vi "Add SR Popup.vi"(8 "error in":errorcluster, 9 "Monitor":u16) -> (0 "error out":errorcluster, 2 "New SR?":bool, 3 "SR array out":i32[](array[numeric]))   [LabVIEW 2018]
uses:
  <vilib>/Utility/miscctls.llb/LVPointTypeDef.ctl
panel:
  in  "Close":bool
  in  "Add SR":bool
  in  "SR to Add":string
  # "Enter SR number(s) seperated by commas\n and press \"Add SRs\" to add it to the list"
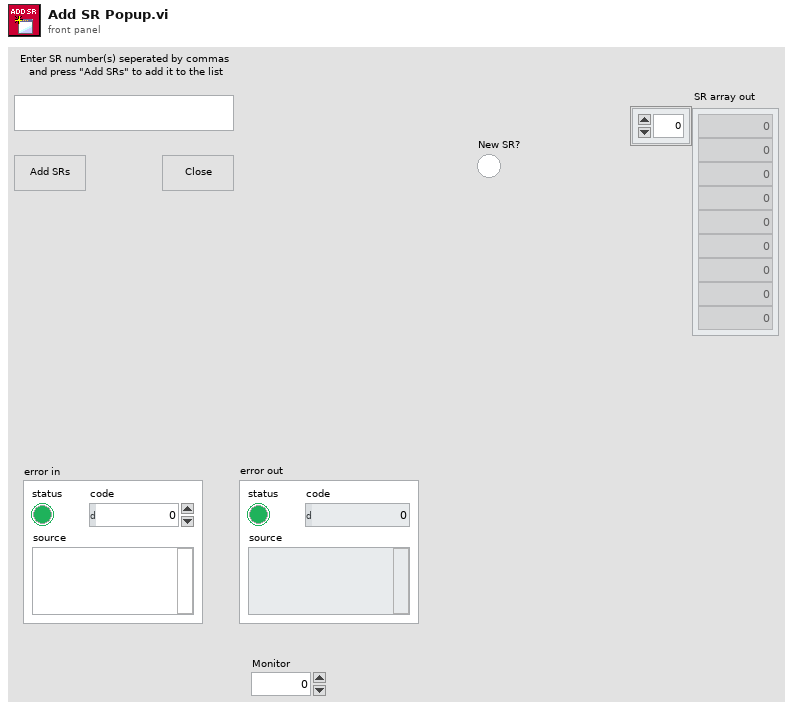
[diagram p1: front panel]
types:
  T1 = typedef "LVPointTypeDef.ctl" = cluster{"Horizontal":i16, "Vertical":i16}
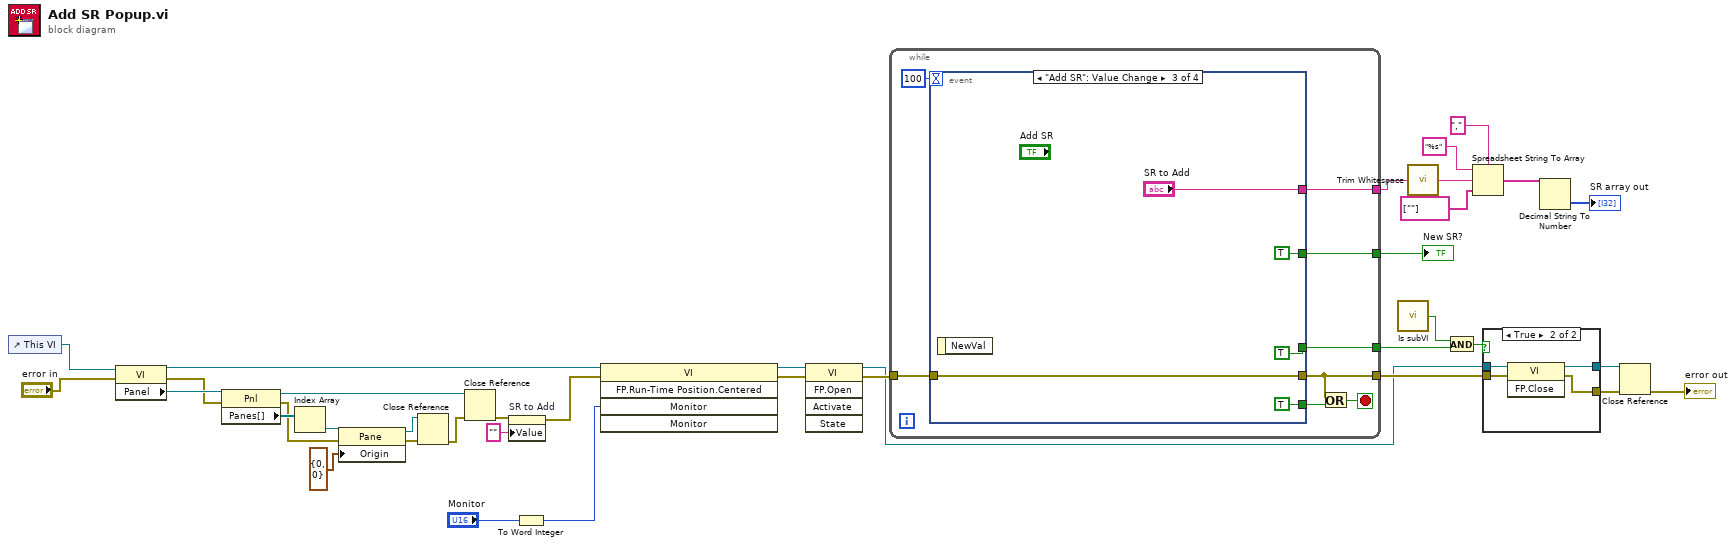
[diagram p0: block diagram]
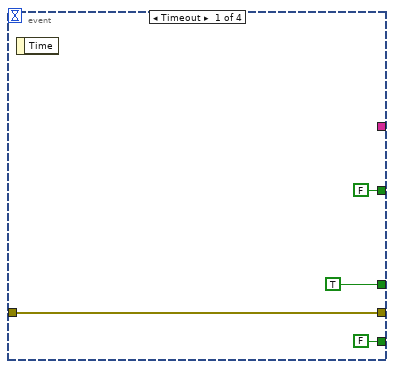
[diagram p3: hidden frame]
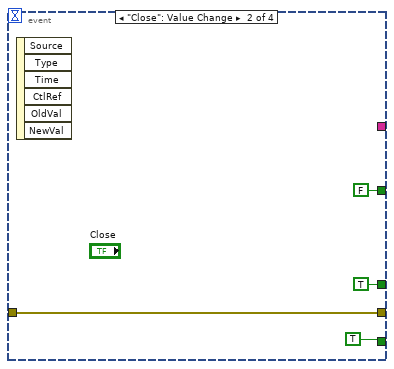
[diagram p4: hidden frame]
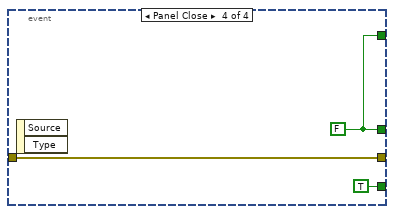
[diagram p5: hidden frame]
diagram:
  n1 = control-ref of="This VI"() -> (w12:refnum<vi>)
  n2 = property class="VI"(reference=w12, error in="error in") -> (reference out=w1:refnum<vi>, error out=w13:errorcluster, "Panel"=w14:refnum<vi>)
  n3 = property class="Pnl"(reference=w14, error in=w13) -> (reference out=w15:refnum<vi>, error out=w20:errorcluster, "Panes[]"=w22:refnum<vi>[])
  n4 = Index Array(array=w22) -> (element=w21:refnum<vi>)  [unwired: 1 in]
  n5 = property class="Pane"(reference=w21, error in=w20, "Origin"=T1 {"Horizontal"=0, "Vertical"=0}) -> (reference out=w18:refnum<vi>, error out=w17:errorcluster)
  n6 = Close Reference(reference=w18, error in (no error)=w17) -> (error out=w16:errorcluster)
  n7 = Close Reference(reference=w15, error in (no error)=w16) -> (error out=w8:errorcluster)
  n8 = property on="SR to Add" class="Str"(error in=w8, "Value"="" ("SR to Add")) -> (error out=w2:errorcluster)  [unwired: 1 in, 1 out]
  n9 = To Word Integer(number="Monitor") -> (16bit integer=w3:i16)
  n10 = invoke class="VI" method="FP.Run-Time Position.Centered"(reference=w1, error in=w2, "Monitor"=w3) -> (reference out=w6:refnum<vi>, error out=w5:errorcluster)  [unwired: 2 in, 3 out]
  n11 = invoke class="VI" method="FP.Open"(reference=w6, error in=w5) -> (reference out=w9:refnum<vi>, error out=w10:errorcluster)  [unwired: 3 in, 3 out]
  n12 = while {
    tunnel: w10 -> [w43]
    tunnel: [w41] -> w37
    tunnel: [w44] -> w24
    tunnel: [w39] -> w33
    tunnel: [w38] -> w31
    stop <- w42 stop-if-true
    n13 = event shown="[2] \"Add SR\": Value Change" {
      selector: _ -> [_ _ _ _]
      dyn-events: _ -> [_ _ _ _]
      timeout: 100 -> [_ _ _ _]
      tunnel: w43 -> [w48 w51 w58 w61]
      tunnel: [w48 w51 w58 w61] -> w41
      tunnel: [TRUE TRUE TRUE w59] -> w44
      tunnel: [FALSE TRUE TRUE TRUE] -> w40
      tunnel: [FALSE FALSE TRUE w59] -> w39
      tunnel: [_ _ "SR to Add" _] -> w38
      event Timeout {
        n14 = event-data() -> ()  [unwired: 1 in, 1 out]
      }
      event "Close": Value Change {
        n15 = event-data() -> ()  [unwired: 1 in, 6 out]
      }
      event "Add SR": Value Change {
        n16 = event-data() -> ()  [unwired: 1 in, 1 out]
      }
      event Panel Close {
        w59 = FALSE
        n17 = event-data() -> ()  [unwired: 1 in, 2 out]
      }
    }
    n18 = Or(x=w41, y=w40) -> (x .or. y?=w42:bool)
  }
  "New SR?" <- w33
  n19 = call "Is subVI.vi"() -> ("Is subVI?"=w23:bool)  [unwired: 1 in]
  n20 = call <vilib>:"Trim Whitespace.vi"("string"=w31) -> ("trimmed string"=w30:string)  [unwired: 1 in]
  n21 = And(x=w23, y=w24) -> (x .and. y?=w25:bool)
  n22 = Spreadsheet String To Array(delimiter (Tab)=",", format string="%s", spreadsheet string=w30, array type (2D Dbl)=string[] [""]) -> (array=w27:string[])
  n23 = case shown="True" w25 {
    tunnel: w9 -> [w63 w67]
    tunnel: w37 -> [w62 w66]
    tunnel: [w63 w65] -> w36
    tunnel: [w62 w64] -> w35
    frame False {
    }
    frame True {
      n24 = invoke class="VI" method="FP.Close"(reference=w67, error in=w66) -> (reference out=w65:refnum<vi>, error out=w64:errorcluster)  [unwired: 1 in, 1 out]
    }
  }
  n25 = Decimal String To Number(string=w27) -> (number=→"SR array out":i32[])  [unwired: 2 in, 1 out]
  n26 = Close Reference(reference=w36, error in (no error)=w35) -> (error out=→"error out":errorcluster)
